vi "Get SD Normal Mode Channels.vi"(8 "error in (no error)":errorcluster, 11 "9402 in":refnum<class "9402.lvclass">) -> (0 "error out":errorcluster, 1 "Channels":T2, 2 "Channel Names":string[](array[string]), 3 "9402 out":refnum<class "9402.lvclass">, 4 "Type":T1)   [LabVIEW 2019, in "Modules.lvlib" / "9402.lvclass"]
uses:
  9402.lvclass
  RSI Module/Channels.ctl
  RSI Module/Channel Type.ctl
  <vilib>/NI VeriStand/Custom Device API/Custom Device Channel Type.ctl
  9402.lvclass/9402.ctl
  RSI Module/RSI Module.lvclass
  <vilib>/NI VeriStand/Custom Device API/Custom Device API.lvlib
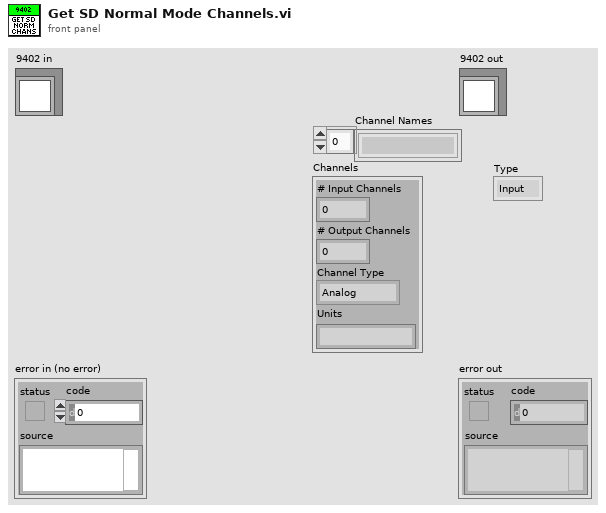
[diagram p1: front panel]
types:
  T1 = typedef "Custom Device API.lvlib/Custom Device Channel Type.ctl" = enum16{"Input", "Output"}
  T2 = typedef "Modules.lvlib/RSI Module.lvclass/Channels.ctl" = cluster{"# Input Channels":i32, "# Output Channels":i32, "Channel Type":T3, "Units":string}
  T3 = typedef "Modules.lvlib/RSI Module.lvclass/Channel Type.ctl" = enum16{"Analog", "Digital"}
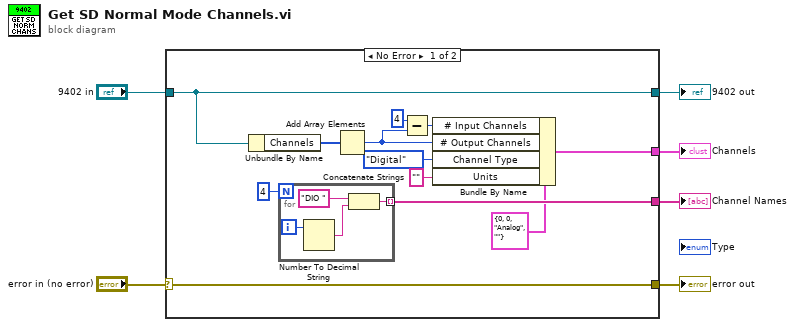
[diagram p0: block diagram]
diagram:
  n1 = case shown="No Error" "error in (no error)" {
    selector: "error in (no error)" -> [w16 w24]
    tunnel: [w16 w24] -> w1
    tunnel: "9402 in" -> [w15 w23]
    tunnel: [w15 w23] -> w4
    tunnel: [w17 _] -> w2
    tunnel: [w9 _] -> w3
    frame No Error {
      n2 = Unbundle By Name(w15) -> ("Channels"=w8:u32[])
      n3 = for {
        N: 4 -> [_]
        tunnel: [w19] -> w17 mode=indexing
        i -> [w22]
        n4 = Number To Decimal String(number=w22) -> (decimal integer string=w20:string)  [unwired: 1 in]
        n5 = Concatenate Strings("DIO ", w20) -> (w19:string)
      }
      n6 = Add Array Elements(numeric array=w8) -> (sum=w7:u32)
      n7 = Subtract(x=u32 4 ("y"), y=w7) -> (x-y=w13:u32)
      n8 = Bundle By Name(cluster=T2 {"# Input Channels"=0, "# Output Channels"=0, "Channel Type"=enum."Analog", "Units"=""} ("Channels"), "# Input Channels"=w13, "# Output Channels"=w7, "Channel Type"=Channel_Type."Digital", "Units"="") -> (w9:T2)
    }
    frame Error {
    }
  }
  "error out" <- w1
  "9402 out" <- w4
  "Channel Names" <- w2
  "Channels" <- w3
